vi "Fail If Error.vi"(7 "Description":string, 8 "error in (no error)":errorcluster, 10 "Assert error":errorcluster, 11 "LUnit Test Case In":refnum<class "LUnit Test Case.lvclass">) -> (0 "error out":errorcluster, 3 "LUnit Test Case Out":refnum<class "LUnit Test Case.lvclass">)   [LabVIEW 2020, in "LUnit Test Case.lvclass"]
doc: "Generates a fail result for the calling test method if the inputs contains an error with status \"True\". A description may be provided to the result."
uses:
  LUnit Test Case.lvclass
  Core/Result/Type.ctl
  LUnit Test Case.lvclass/LUnit Test Case.ctl
  Core/Result/Result.lvlib
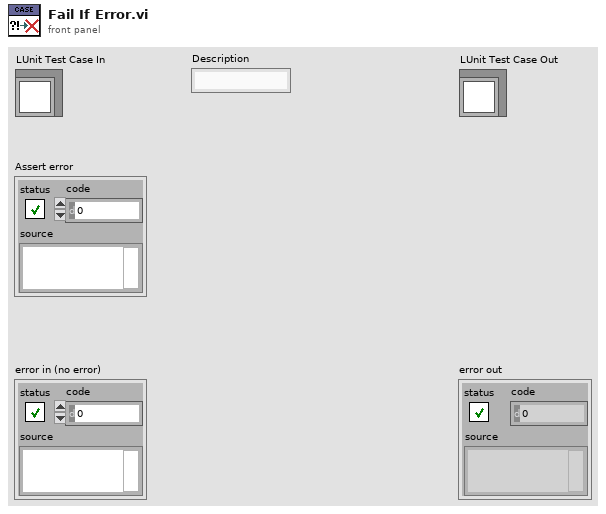
[diagram p1: front panel]
types:
  T1 = typedef "Result.lvlib/Type.ctl" = enum16{"Test Case", "Test Suite", "Test Run", "Pass", "Fail", "Skip", "Pass if", "Fail if", "Pass if Error", "Fail if Error", "Pass if Equal", "Fail if Equal"}
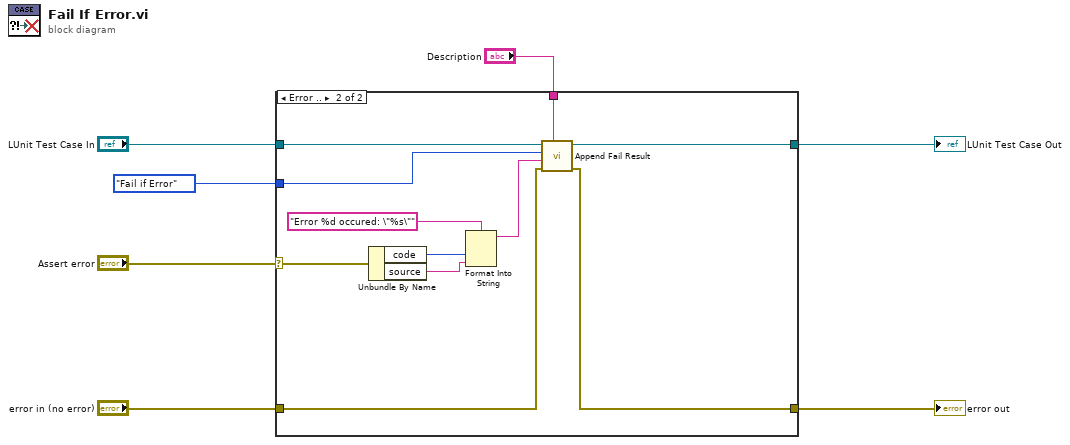
[diagram p0: block diagram]
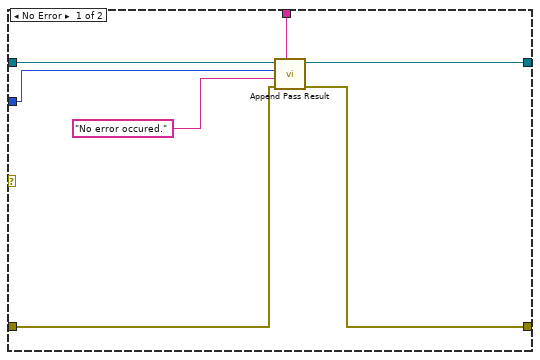
[diagram p2: hidden frame]
diagram:
  n1 = case shown="Error .." "Assert error" {
    selector: "Assert error" -> [_ w22]
    tunnel: "LUnit Test Case In" -> [w14 w25]
    tunnel: [w13 w24] -> w5
    tunnel: [w12 w23] -> w4
    tunnel: "Description" -> [w11 w19]
    tunnel: "error in (no error)" -> [w9 w16]
    tunnel: Type."Fail if Error" ("Result Type") -> [w8 w15]
    frame No Error {
      n2 = call "Append Pass Result.vi"("Description"=w11, "error in (no error)"=w9, "Message"="No error occured.", "Result Type"=w8, "LUnit Test Case In"=w14) -> ("error out"=w12:errorcluster, "LUnit Test Case Out"=w13:refnum<class "LUnit Test Case.lvclass">)  [unwired: 5 in]
    }
    frame Error {
      n3 = Unbundle By Name(w22) -> ("code"=w18:i32, "source"=w17:string)
      n4 = Format Into String(format string="Error %d occured: \"%s\"", w18, w17) -> (resulting string=w21:string)  [unwired: 2 in, 1 out]
      n5 = call "Append Fail Result.vi"("Description"=w19, "error in (no error)"=w16, "Message"=w21, "Result Type"=w15, "LUnit Test Case In"=w25) -> ("error out"=w23:errorcluster, "LUnit Test Case Out"=w24:refnum<class "LUnit Test Case.lvclass">)  [unwired: 5 in]
    }
  }
  "error out" <- w4
  "LUnit Test Case Out" <- w5
